vi "StringMonitorUserData.vi"() -> ()   [LabVIEW 2016, in "StringIntelliSense.lvlib" / "IntelliSenseStringControl.lvclass"]
uses:
  IntelliSenseStringControl.lvclass
panel:
  in  "IntelliSense String []":refnum<class "IntelliSenseStringControl.lvclass">[](array[class])
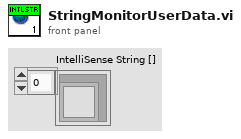
[diagram p1: front panel]
diagram:
